vi "Initialize.vi"(6 "type":string=".csv", 8 "error in (no error)":errorcluster, 9 "File name":string, 10 "Path":path, 11 "Save as csv in":refnum<class "Save as csv.lvclass">) -> (0 "error out":errorcluster, 3 "Save as csv out":refnum<class "Save as csv.lvclass">)   [LabVIEW 2020, in "Save as csv.lvclass"]
uses:
  Save as csv.lvclass
  Saving OO.lvclass
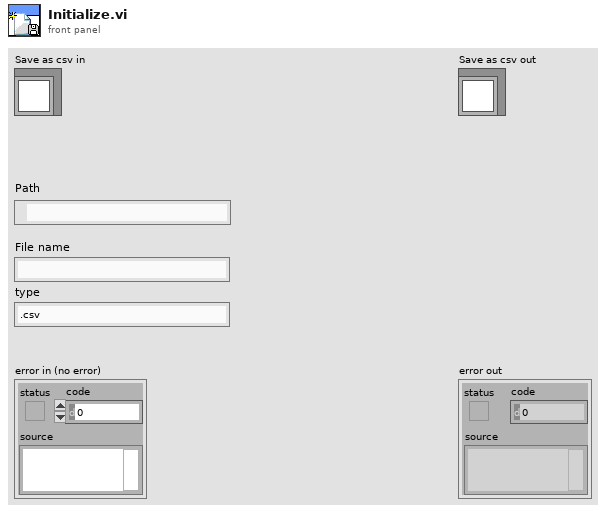
[diagram p1: front panel]
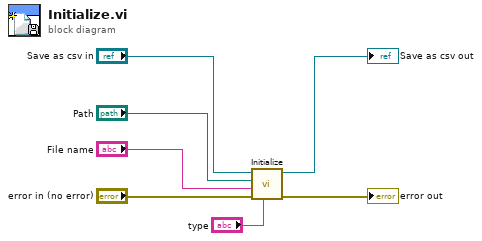
[diagram p0: block diagram]
diagram:
  n1 = call-parent "Initialize.vi"("type"="type", "error in (no error)"="error in (no error)", "File name"="File name", "Path"="Path", "Saving OO in"="Save as csv in") -> ("error out"=→"error out":errorcluster, "Saving OO out"=→"Save as csv out":refnum<class "Save as csv.lvclass">)  [unwired: 5 in]
